vi "DDSSequence_STPramp.vi"(6 "Freqeuncy (MHz)":dbl[][](array[numeric]), 7 "Power":dbl[][](array[numeric]), 9 "Channels":T2(ring), 10 "Duration (ms)":dbl[][](array[numeric]), 11 "No of  active time blocks":dbl) -> (3 "appended instruction string":string)   [LabVIEW 2016]
panel:
  out "x/y":dbl
  in  "Ramp duration (us)":dbl=40.0 format="%#_6f"
  out "Step seperation (us)":dbl=0.4
  in  "Step Size":dbl=0.01 format="%#_6f"
  in  "Max Value":dbl=1.0 format="%#_13g"
  in  "Min Value":dbl format="%#_6f"
  in  "Ramp type":enum32{"Frequency", "Phase", "Amplitude"}(ring)=enum."Amplitude"
  in  "Ramp trigger source":T1(ring)=enum."BNC_IN_A_RISING"
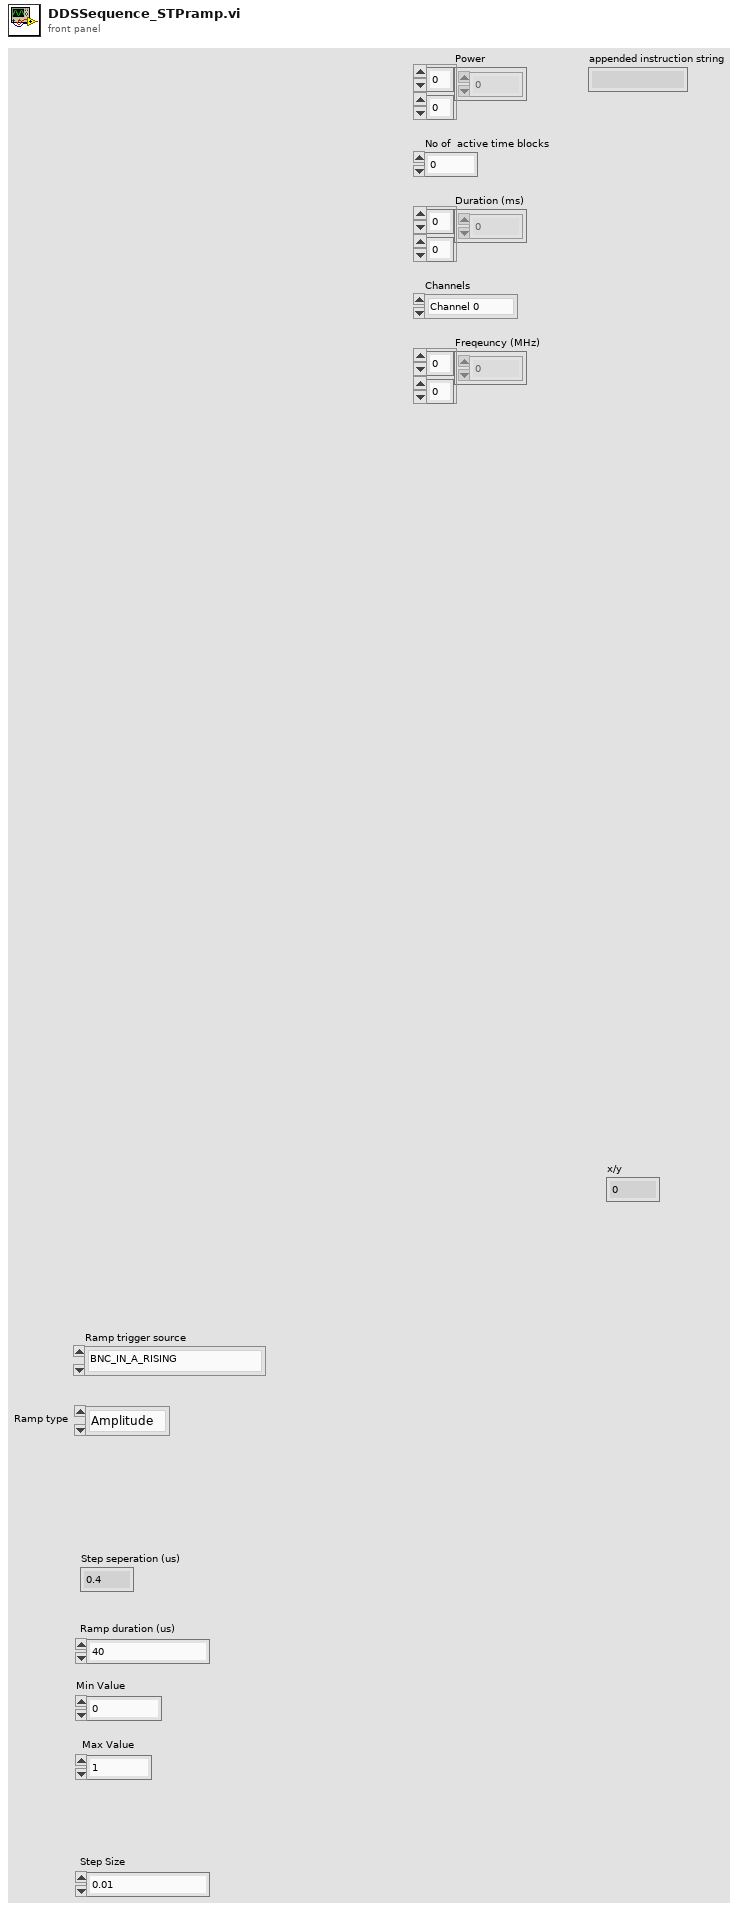
[diagram p1: front panel]
types:
  T1 = enum32{"O_RAMP_SWP_OVR", "RAM_SWP_OVR", "O_DROVER", "DROVER", "O_SPI_FIFO_EV1", "SPI_FIFO_EV1", "O_SPI_FIFO_EV0", "SPI_FIFO_EV0", "O_SPI_FIFO_FLUSHED", "SPI_FIFO_FLUSHED", "BNC_IN_B_LEVEL", "BNC_IN_B_FALLING", "BNC_IN_B_RISING", "BNC_IN_A_LEVEL", "BNC_IN_A_FALLING", "BNC_IN_A_RISING", "ALL_SPI_FIFOS_FLUSHED", "NONE"}
  T2 = enum32{"Channel 0", "Channel 1", "Both channels"}
  T3 = cluster{"Enable ASF from STP (F)":bool, "Digital ramp enable (F)":bool, "Digital ramp no-dwell high (F)":bool, "Digital ramp no-dwell low (F)":bool, "Matched latency enable (T)":bool, "Parallel data port enable (F)":bool}
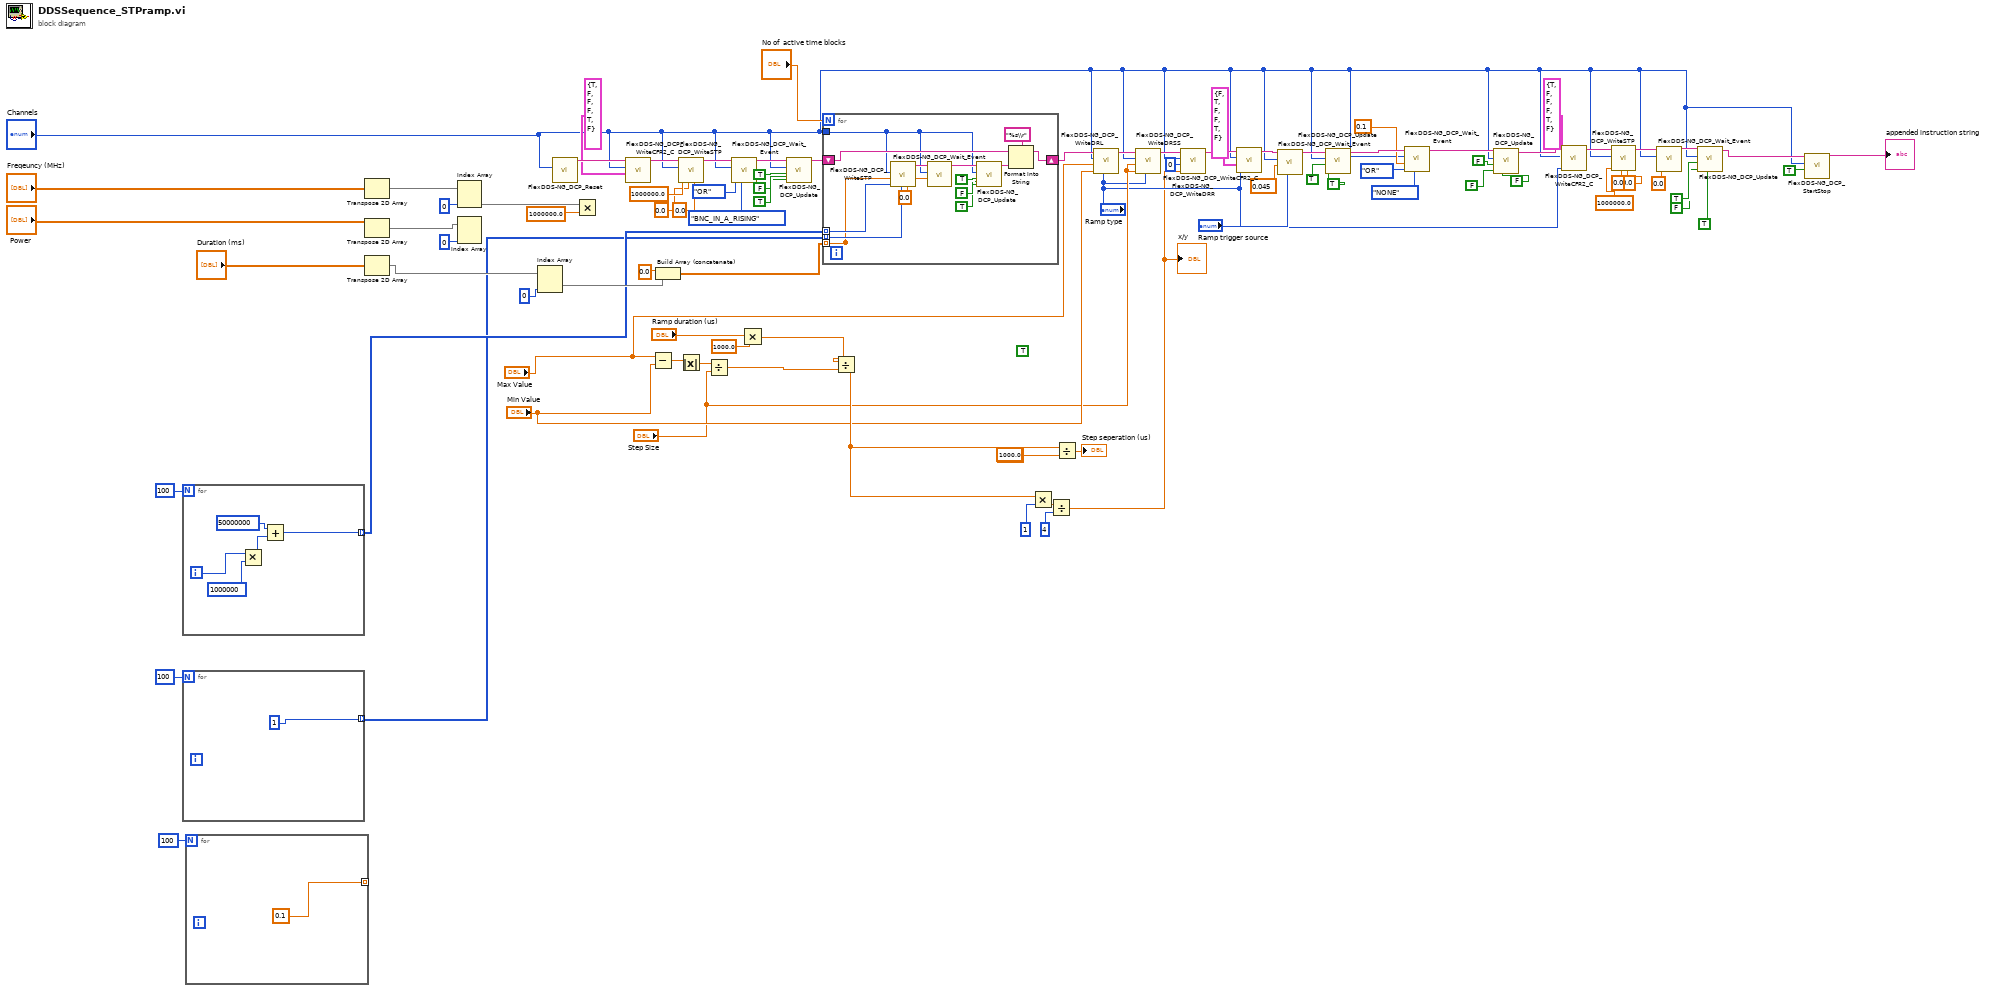
[diagram p0: block diagram]
diagram:
  (unwired) 1000.0 ("x/y")
  (unwired) TRUE ("DRCTL(true=+, false=-) 2")
  n1 = for {
    N: 100 -> [_]
    tunnel: [w88] -> w4 mode=indexing
    i -> [w92]
    n2 = Multiply(x=w92, y=1000000) -> (x*y=w89:i32)
    n3 = Add(x=50000000, y=w89) -> (x+y=w88:i32)
  }
  n4 = for {
    N: 100 -> [_]
    tunnel: [1 ("y")] -> w2 mode=indexing
    i -> [w94]
  }
  n5 = for {
    N: 100 -> [_]
    tunnel: [0.1 ("x/y")] -> _ mode=indexing
    i -> [w96]
  }
  n6 = Transpose 2D Array(2D array="Freqeuncy (MHz)") -> (transposed array=w77:dbl[][])
  n7 = Transpose 2D Array(2D array="Power") -> (transposed array=w75:dbl[][])
  n8 = Transpose 2D Array(2D array="Duration (ms)") -> (transposed array=w87:dbl[][])
  n9 = Index Array(array=w77, index (col)=0 ("index (row)")) -> (element=w79:dbl[])  [unwired: 1 in]
  n10 = Index Array(array=w75, index (col)=0 ("index (row)")) -> ()  [unwired: 1 in, 1 out]
  n11 = Index Array(array=w87, index (col)=0 ("index (row)")) -> (element=w84:dbl[])  [unwired: 1 in]
  n12 = call "FlexDDS-NG_DCP_Reset.vi"("Channels"="Channels") -> ("appended instruction string"=w61:string)  [unwired: 10 in]
  n13 = Multiply(x=w79, y=1000000.0 ("frequency Hz (0..400M)")) -> ()  [unwired: 1 out]
  n14 = call "FlexDDS-NG_DCP_WriteCFR2_C.vi"("CFR2 bits"=T3 {"Enable ASF from STP (F)"=TRUE, "Digital ramp enable (F)"=FALSE, "Digital ramp no-dwell high (F)"=FALSE, "Digital ramp no-dwell low (F)"=FALSE, "Matched latency enable (T)"=TRUE, "Parallel data port enable (F)"=FALSE} ("CFR2 bits 2"), "Channels"="Channels", "initial instruction string"=w61) -> ("appended instruction string"=w60:string)  [unwired: 8 in]
  n15 = Subtract(x="Max Value", y="Min Value") -> (x-y=w18:dbl)
  n16 = Build Array (concatenate)(0.0 ("phase degrees (0..360)"), w84) -> (w85:dbl[])
  n17 = call "FlexDDS-NG_DCP_WriteSTP.vi"("phase degrees (0..360)"=0.0, "amplitude (0..1)"=0.0, "frequency Hz (0..400M)"=1000000.0, "Channels"="Channels", "initial instruction string"=w60) -> ("appended instruction string"=w66:string)  [unwired: 6 in]
  n18 = Absolute Value(x=w18) -> (abs(x)=w17:dbl)
  n19 = Divide(x=w17, y="Step Size") -> (x/y=w22:dbl)
  n20 = call "FlexDDS-NG_DCP_Wait_Event.vi"("Event 1"=T1."BNC_IN_A_RISING", "AND/OR"=enum32{"AND", "OR"}."OR", "Channels in"="Channels", "appended instruction string in"=w66) -> ("appended instruction string"=w65:string)  [unwired: 7 in]
  n21 = Multiply(x="Ramp duration (us)", y=1000.0) -> (x*y=w12:dbl)
  n22 = call "FlexDDS-NG_DCP_Update.vi"("ONLY IO_UPDATE"=TRUE, "DRCTL(true=+, false=-)"=FALSE ("DRCTL(true=+, false=-) 2"), "IO_UPDATE(true=u, false = '')"=TRUE ("IO_UPDATE(true=u, false = '')  2"), "Channels"="Channels", "appended instruction string in"=w65) -> ("appended instruction string out"=w71:string)  [unwired: 6 in]
  n23 = for {
    N: "No of  active time blocks" -> [_]
    shift-right: [w102] -> w29
    shift-left: w71 -> [w103]
    tunnel: w2 -> [w100] mode=indexing
    tunnel: "Channels" -> [w99]
    tunnel: w85 -> [w97] mode=indexing
    tunnel: w4 -> [w98] mode=indexing
    tunnel: [w97] -> _ mode=indexing
    n24 = call "FlexDDS-NG_DCP_WriteSTP.vi"("phase degrees (0..360)"=0.0, "amplitude (0..1)"=w100, "frequency Hz (0..400M)"=w98, "Channels"=w99) -> ("appended instruction string"=w105:string)  [unwired: 7 in]
    n25 = call "FlexDDS-NG_DCP_Wait_Event.vi"("waiting time [ms]"=w97, "Channels in"=w99, "appended instruction string in"=w105) -> ("appended instruction string"=w106:string)  [unwired: 8 in]
    n26 = call "FlexDDS-NG_DCP_Update.vi"("ONLY IO_UPDATE"=TRUE, "DRCTL(true=+, false=-)"=FALSE ("DRCTL(true=+, false=-) 2"), "IO_UPDATE(true=u, false = '')"=TRUE ("IO_UPDATE(true=u, false = '')  2"), "Channels"=w99, "appended instruction string in"=w106) -> ("appended instruction string out"=w101:string)  [unwired: 6 in]
    n27 = Format Into String(format string="%s\\r", initial string=w103, w101) -> (resulting string=w102:string)  [unwired: 1 in, 1 out]
  }
  n28 = Divide(x=w12, y=w22) -> (x/y=w21:dbl)
  n29 = Multiply(x=w21, y=u16 1) -> (x*y=w24:dbl)
  n30 = Divide(x=w24, y=u16 4) -> (x/y=w7:dbl)
  "x/y" <- w7
  n31 = Divide(x=w21, y=1000.0 ("x/y")) -> (x/y=→"Step seperation (us)":dbl)
  n32 = call "FlexDDS-NG_DCP_WriteDRL.vi"("Ramp type"="Ramp type", "low limit"="Min Value", "high limit"="Max Value", "Channels"="Channels", "initial instruction string"=w29) -> ("appended instruction string"=w56:string)  [unwired: 6 in]
  n33 = call "FlexDDS-NG_DCP_WriteDRSS.vi"("Ramp type"="Ramp type", "increment step size"="Step Size", "decrement step size"="Step Size", "Channels"="Channels", "initial instruction string"=w56) -> ("appended instruction string"=w55:string)  [unwired: 6 in]
  n34 = call "FlexDDS-NG_DCP_WriteDRR.vi"("digital ramp positive slope rate"=w7, "digital ramp negative slope rate"=u16 0, "Channels"="Channels", "initial instruction string"=w55) -> ("appended instruction string"=w54:string)  [unwired: 7 in]
  n35 = call "FlexDDS-NG_DCP_WriteCFR2_C.vi"("Digital ramp destination"="Ramp type", "CFR2 bits"=T3 {"Enable ASF from STP (F)"=FALSE, "Digital ramp enable (F)"=TRUE, "Digital ramp no-dwell high (F)"=FALSE, "Digital ramp no-dwell low (F)"=FALSE, "Matched latency enable (T)"=TRUE, "Parallel data port enable (F)"=FALSE}, "Channels"="Channels", "initial instruction string"=w54) -> ("appended instruction string"=w50:string)  [unwired: 7 in]
  n36 = call "FlexDDS-NG_DCP_Wait_Event.vi"("Event 1"="Ramp trigger source", "waiting time [ms]"=0.045, "Channels in"="Channels", "appended instruction string in"=w50) -> ("appended instruction string"=w49:string)  [unwired: 7 in]
  n37 = call "FlexDDS-NG_DCP_Update.vi"("DRCTL(true=+, false=-)"=TRUE, "IO_UPDATE(true=u, false = '')"=TRUE, "Channels"="Channels", "appended instruction string in"=w49) -> ("appended instruction string out"=w44:string)  [unwired: 7 in]
  n38 = call "FlexDDS-NG_DCP_Wait_Event.vi"("Event 1"=T1."NONE", "AND/OR"=enum32{"AND", "OR"}."OR", "waiting time [ms]"=0.1 ("y"), "Channels in"="Channels", "appended instruction string in"=w44) -> ("appended instruction string"=w32:string)  [unwired: 6 in]
  n39 = call "FlexDDS-NG_DCP_Update.vi"("ONLY IO_UPDATE"=FALSE, "DRCTL(true=+, false=-)"=FALSE ("DRCTL(true=+, false=-) 2"), "IO_UPDATE(true=u, false = '')"=FALSE ("IO_UPDATE(true=u, false = '')  2"), "Channels"="Channels", "appended instruction string in"=w32) -> ("appended instruction string out"=w33:string)  [unwired: 6 in]
  n40 = call "FlexDDS-NG_DCP_WriteCFR2_C.vi"("Digital ramp destination"="Ramp type", "CFR2 bits"=T3 {"Enable ASF from STP (F)"=TRUE, "Digital ramp enable (F)"=FALSE, "Digital ramp no-dwell high (F)"=FALSE, "Digital ramp no-dwell low (F)"=FALSE, "Matched latency enable (T)"=TRUE, "Parallel data port enable (F)"=FALSE}, "Channels"="Channels", "initial instruction string"=w33) -> ("appended instruction string"=w38:string)  [unwired: 7 in]
  n41 = call "FlexDDS-NG_DCP_WriteSTP.vi"("phase degrees (0..360)"=0.0, "amplitude (0..1)"=0.0, "frequency Hz (0..400M)"=1000000.0, "Channels"="Channels", "initial instruction string"=w38) -> ("appended instruction string"=w37:string)  [unwired: 6 in]
  n42 = call "FlexDDS-NG_DCP_Wait_Event.vi"("waiting time [ms]"=0.0, "Channels in"="Channels", "appended instruction string in"=w37) -> ("appended instruction string"=w36:string)  [unwired: 8 in]
  n43 = call "FlexDDS-NG_DCP_Update.vi"("ONLY IO_UPDATE"=TRUE, "DRCTL(true=+, false=-)"=FALSE ("DRCTL(true=+, false=-) 2"), "IO_UPDATE(true=u, false = '')"=TRUE ("IO_UPDATE(true=u, false = '')  2"), "Channels"="Channels", "appended instruction string in"=w36) -> ("appended instruction string out"=w28:string)  [unwired: 6 in]
  n44 = call "FlexDDS-NG_DCP_StartStop.vi"("start (T) stop (F)"=TRUE, "Channels"="Channels", "initial instruction string"=w28) -> ("appended instruction string"=→"appended instruction string":string)  [unwired: 8 in]
